vi "FPGAztrajectoryAdjustable.vi"(1 "z step size derived":u16, 2 "Vz min (bits)":i16, 3 "z/intensity memory address":u16) -> (0 "Z trajectory":i16)   [LabVIEW 2010]
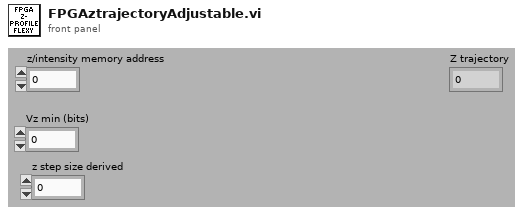
[diagram p1: front panel]
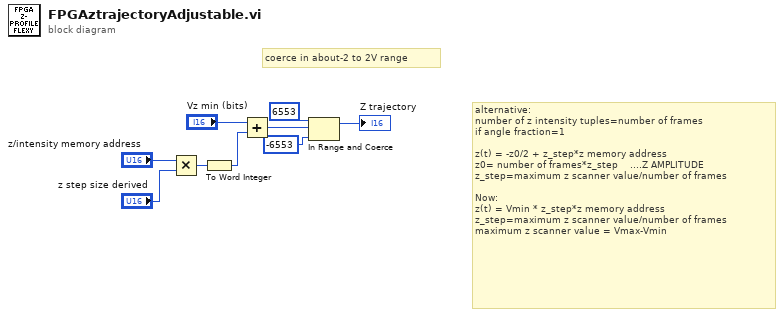
[diagram p0: block diagram]
diagram:
  # "alternative:\nnumber of z intensity tuples=number of frames\nif angle fraction=1\n\nz(t) = -z0/2 + z_step*z memory address\nz0= number of frames*z_step    ....Z AMPLITUDE\nz_step=maximum z scanner value/number of frames\n\nNow:\nz(t) = Vmin * z_step*z memory address\nz_step=maximum z scanner value/number of frames\nmaximum z scanner value = Vmax-Vmin"
  # "coerce in about-2 to 2V range"
  n1 = Multiply(x="z/intensity memory address", y="z step size derived") -> (x*y=w4:u16)
  n2 = To Word Integer(number=w4) -> (16bit integer=w5:i16)
  n3 = Add(x="Vz min (bits)", y=w5) -> (x+y=w8:i16)
  n4 = In Range and Coerce(upper limit=i16 6553, x=w8, lower limit=i16 -6553) -> (coerced(x)=→"Z trajectory":i16)  [unwired: 1 out]
